vi "Stop Core.vi"(10 "final error code":i32, 11 "Child Actor in":refnum<class "Child Actor.lvclass">) -> (3 "Child Actor out":refnum<class "Child Actor.lvclass">)   [LabVIEW 2012, in "Child Actor.lvclass"]
doc: "(<B>Filename</B>: Actor Framework.lvlib:Actor.lvclass:Stop Core.vi)\n\nDefines what the actor does before it stops. Use the <B>final error code</B> input to determine whether the actor shut down in response to an error.\n\nBy default, this method does nothing. A descendant class may override it to define behavior, such as shutting down any processes the actor initiated in its override of the Actor Core method."
uses:
  Child Actor.lvclass
  <vilib>/ActorFramework/Actor/Actor.lvclass
  Child Actor.lvclass/Child Actor.ctl
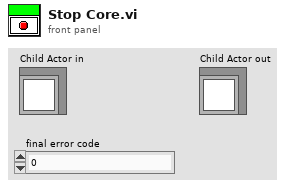
[diagram p1: front panel]
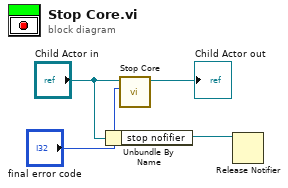
[diagram p0: block diagram]
diagram:
  n1 = Unbundle By Name("Child Actor in") -> ("stop nofifier"=w1:refnum<notifier>)
  n2 = call-parent "Stop Core.vi"("final error code"="final error code", "Actor in"="Child Actor in") -> ("Actor out"=→"Child Actor out":refnum<class "Child Actor.lvclass">)  [unwired: 9 in]
  n3 = Release Notifier(notifier=w1) -> ()  [unwired: 2 in, 3 out]
